vi "GlobalRECnew.vi"() -> ()   [LabVIEW 2020]
panel:
  out "Boolean":bool
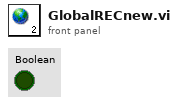
[diagram p1: front panel]
diagram:
